vi "Write Test Report.vi"(10 "Test Report":refnum<class "Test Report.lvclass">, 11 "Basic Test Manager":refnum<class "Basic Test Manager.lvclass">) -> (3 "Basic Test Manager":refnum<class "Basic Test Manager.lvclass">)   [LabVIEW 2013, in "Caraya.lvlib" / "Basic Test Manager.lvclass"]
uses:
  Basic Test Manager.lvclass
  Test Report/Test Report.lvclass
  Basic Test Manager.lvclass/Basic Test Manager.ctl
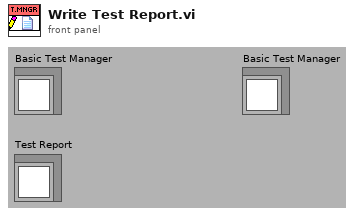
[diagram p1: front panel]
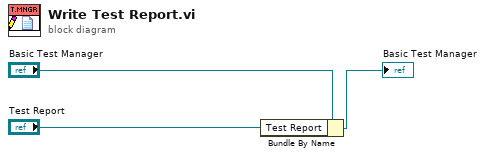
[diagram p0: block diagram]
diagram:
  n1 = Bundle By Name(cluster="Basic Test Manager", "Test Report"="Test Report") -> (→"Basic Test Manager":refnum<class "Basic Test Manager.lvclass">)
